vi "Raw Output to Boolean Output.vi"(10 "Raw Data":u8[](array[numeric])) -> (2 "Output State":bool[](array[boolean]))   [LabVIEW 2018, in "PIOD.lvlib" / "PIOD.lvclass"]
uses:
  PIOD.lvclass
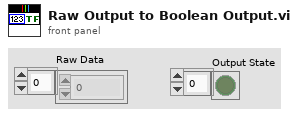
[diagram p1: front panel]
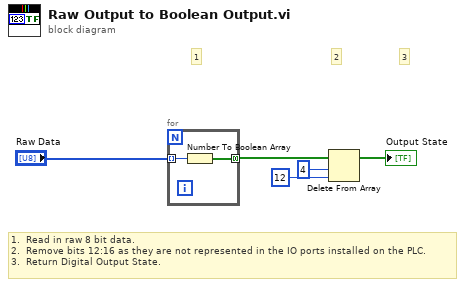
[diagram p0: block diagram]
diagram:
  # "3"
  # "1.  Read in raw 8 bit data.\n2.  Remove bits 12:16 as they are not represented in the IO ports installed on the PLC.\n3.  Return Digital Output State."
  # "2"
  # "1"
  n1 = for {
    tunnel: "Raw Data" -> [w7] mode=indexing
    tunnel: [w6] -> w4 mode=concatenating
    n2 = Number To Boolean Array(number=w7) -> (Boolean array=w6:bool[])
  }
  n3 = Delete From Array(array=w4, length=4, index=12) -> (array with subset deleted=→"Output State":bool[])  [unwired: 1 out]
